vi "Abort Secondary FPGA.vi"() -> ()   [LabVIEW 2022 SP3]
doc: "Author: Scott Hannahs <sth@magnet.fsu.edu>\nCopyright 2018 Florida State University, All rights reserved."
uses:
  <vilib>/userDefined/Silver/nirio_resource_slv.ctl
  <vilib>/FPGAPlugInAG/cRIO-9039/niLvFpga_Open_cRIO-9039.vi
  <vilib>/rvi/interface/common/dynamic/niFpgaDynamicAddResources.vi
  <vilib>/FPGAPlugInAG/Dynamic/niLvFpga_Abort_Dynamic.vi
  <vilib>/FPGAPlugInAG/Dynamic/niLvFpga_Close_Dynamic.vi
  <vilib>/rvi/interface/nirviOpenFPGA/nirviOpenFPGA.xnode
  FPGA Bitfiles/SCHProtection_SCHMPSSecondaryF_SecondaryFPGADig_T6ps523+tyQ.lvbitx
  <vilib>/rvi/interface/nirviMethod/nirviMethod.xnode
  <vilib>/rvi/interface/nirviCloseFPGA/nirviCloseFPGA.xnode
panel:
  out "error out":errorcluster
  in  "resource name":T1="rio://localhost/RIO0"
  in  "error in":errorcluster
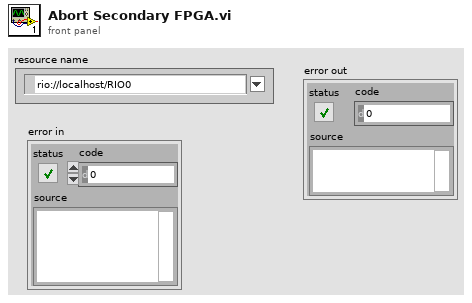
[diagram p1: front panel]
types:
  T1 = typedef "nirio_resource_slv.ctl" = tag
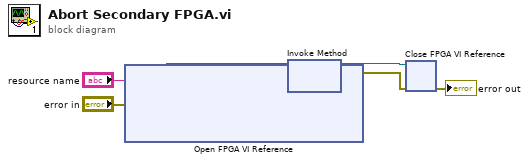
[diagram p0: block diagram]
diagram:
  n1 = xnode "Open FPGA VI Reference"("error in"="error in", "resource name"="resource name") -> ("FPGA VI Reference Out"=w5:refnum<k20>, "error out"=w4:errorcluster)
  n2 = xnode "Invoke Method"("FPGA VI Reference In"=w5, "error in"=w4) -> ("FPGA VI Reference Out"=w3:refnum<k20>, "error out"=w2:errorcluster)
  n3 = xnode "Close FPGA VI Reference"("FPGA VI Reference In"=w3, "error in"=w2) -> ("error out"=→"error out":errorcluster)
